vi "Counter.vi"() -> ()   [LabVIEW 2014]
panel:
  out "self-test message":string
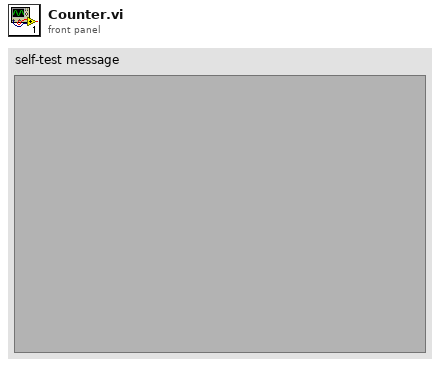
[diagram p1: front panel]
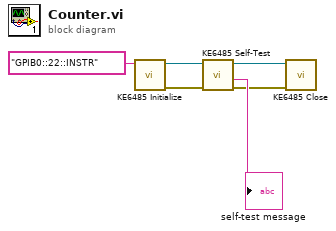
[diagram p0: block diagram]
diagram:
  n1 = call <instrlib>:"KE6485 Initialize.vi"("resource name"="GPIB0::22::INSTR") -> ("error out"=w5:errorcluster, "instrument handle out"=w6:refnum<k15>)  [unwired: 9 in]
  n2 = call <instrlib>:"KE6485 Self-Test.vi"("error in (no error)"=w5, "instrument handle"=w6) -> ("error out"=w1:errorcluster, "self-test message"=→"self-test message":string, "instrument handle out"=w2:refnum<k15>)  [unwired: 6 in, 1 out]
  n3 = call <instrlib>:"KE6485 Close.vi"("error in (no error)"=w1, "instrument handle"=w2) -> ()  [unwired: 9 in, 1 out]
